vi "properties.set.vi"   [LabVIEW 2020, in "type.lvclass"]
uses:
  type.lvclass
  type.lvclass/type.ctl
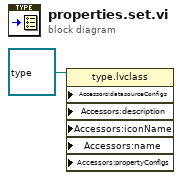
[diagram p0: block diagram]
diagram:
  n1 = property class="type.lvclass" props=["Accessors:datasourceConfigs", "Accessors:description", "Accessors:iconName", "Accessors:name", "Accessors:propertyConfigs"](reference=refnum<class "type.lvclass"> refnum ("type.lvclass")) -> ()  [unwired: 6 in, 2 out]
